vi "CALC_TRAN_TIME_MARK_UNIT.vi"(0 "VISA IN":refnum<visa-resource-name>, 1 "UNIT":string(combo), 5 "error in":errorcluster, 7 "Channel":i32) -> (14 "VISA Out":refnum<visa-resource-name>, 19 "error out":errorcluster)   [LabVIEW 2018, in "PNA-X.lvlib"]
doc: "CALCulate<cnum>:TRANsform:TIME:MARKer:UNIT <char> \n(Read-Write) Specifies the unit of measure for the display of marker distance values. This settings \naffects the display of ALL markers for only the ACTIVE measurement (unless Distance Maker Units \nare coupled using CALC:TRAN:COUP:PAR. \nLearn more about Distance Markers. \nSee Critical Note \nParameters \n<cnum> Channel number of the measurement. There must be a selected measurement \non that channel. If unspecified, <cnum> is set to 1. \n<char> Choose from: \nMETRs \nFEET \nINCHes \nExamples CALC:TRAN:TIME:MARK:UNIT INCH \ncalculate2:transform:time:marker:unit feet \nQuery Syntax CALCulate<cnum>:TRANsform:TIME:MARKer:UNIT? \nReturn Type Character \nDefault METRs"
uses:
  PNA-X.lvlib
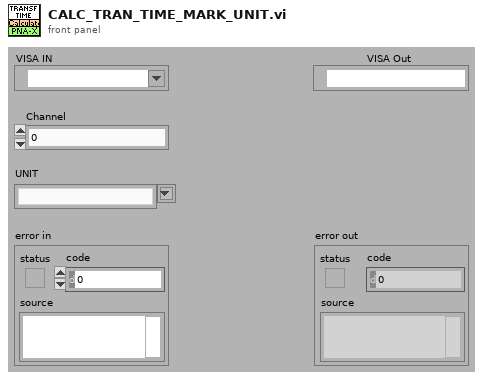
[diagram p1: front panel]
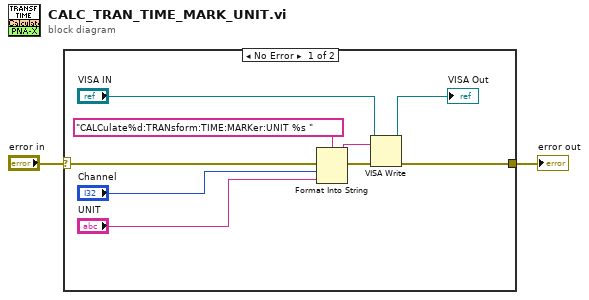
[diagram p0: block diagram]
diagram:
  n1 = case shown="No Error" "error in" {
    selector: "error in" -> [w11 w12]
    tunnel: [w6 w12] -> w1
    frame No Error {
      n2 = Format Into String(format string="CALCulate%d:TRANsform:TIME:MARKer:UNIT %s " ("Cmdline"), error in=w11, "Channel", "UNIT") -> (resulting string=w9:string, error out=w10:errorcluster)  [unwired: 1 in]
      n3 = VISA Write(VISA resource name="VISA IN", write buffer=w9, error in (no error)=w10) -> (VISA resource name out=→"VISA Out":refnum<visa-resource-name>, error out=w6:errorcluster)  [unwired: 1 out]
    }
    frame Error {
    }
  }
  "error out" <- w1
